vi "TDMS to ASCII convertor.vi"(8 "error in":errorcluster, 9 "Group handling":enum16{"One file per group", "Ignore groups"}(ring), 11 "TDMS file path":path) -> (0 "error out":errorcluster, 3 "Generated File Path(s)":path[](array[path]))   [LabVIEW 2016]
uses:
  <vilib>/Utility/file.llb/Write To Spreadsheet File (string).vi
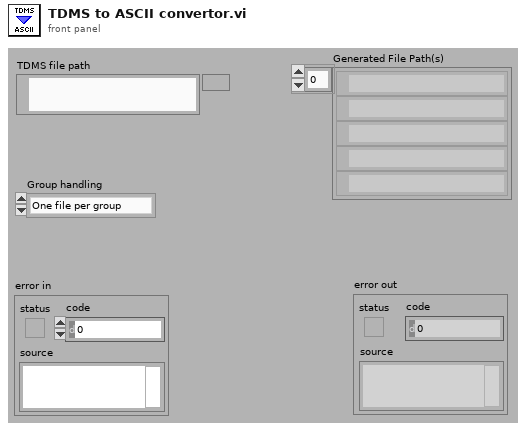
[diagram p1: front panel]
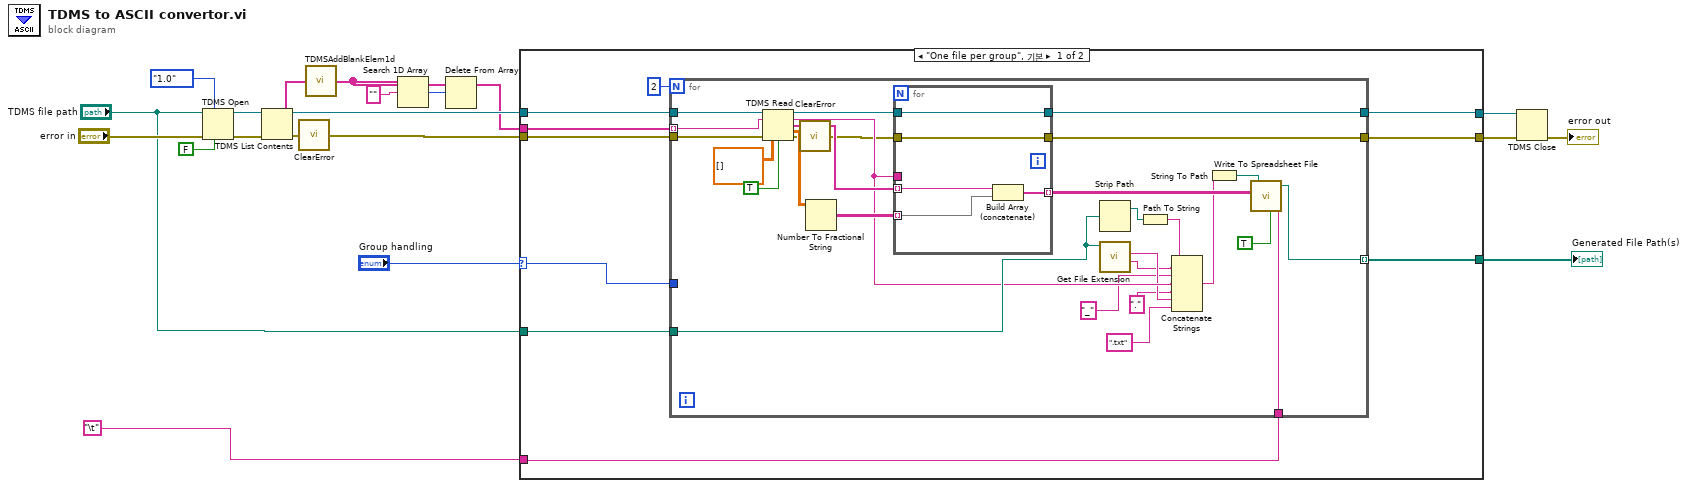
[diagram p0: block diagram]
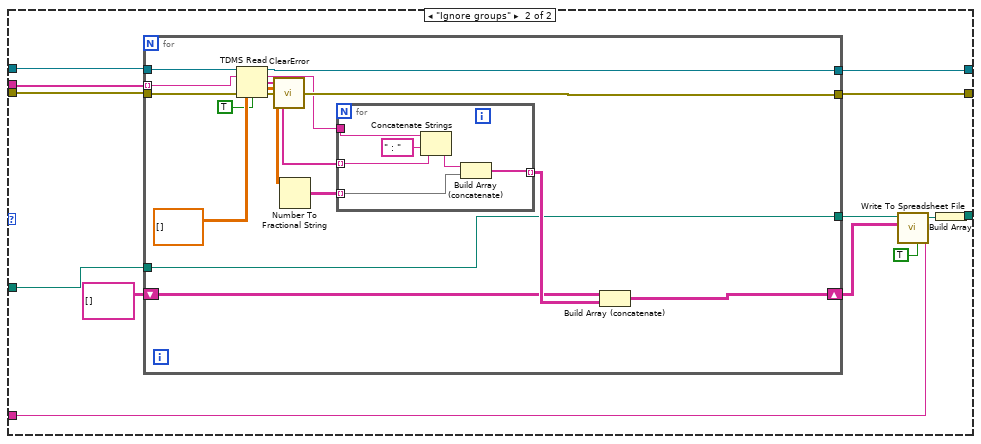
[diagram p2: hidden frame]
diagram:
  n1 = TDMS Open(6:FALSE ("버퍼링 비활성화? (참)"), 7:enum16{"1.0", "2.0"}."1.0" ("파일 포맷 버전(2.0)"), 8:"error in", 11:"TDMS file path") -> (0:w17:errorcluster, 3:w18:refnum<k34>)  [unwired: 3 in]
  n2 = TDMS List Contents(4:w17, 7:w18) -> (0:w1:errorcluster, 2:w4:string[], 3:w16:refnum<k34>)  [unwired: 1 in, 1 out]
  n3 = call <vilib>:"ClearError.vi"("error in (no error)"=w1) -> ("error out"=w15:errorcluster)
  n4 = call <vilib>:"TDMSAddBlankElem1d.vi"("input string array"=w4) -> ("output string array with blank element at the beginning"=w9:string[])
  n5 = Search 1D Array(1D array=w9, element="") -> (index of element=w7:i32)  [unwired: 1 in]
  n6 = Delete From Array(array=w9, index=w7) -> (array with subset deleted=w14:string[])  [unwired: 1 in, 1 out]
  n7 = case shown="\"One file per group\", 기본" "Group handling" {
    selector: "Group handling" -> [w29 _]
    tunnel: "TDMS file path" -> [w30 w73]
    tunnel: [w28 w68] -> w19
    tunnel: w16 -> [w24 w76]
    tunnel: w14 -> [w27 w75]
    tunnel: w15 -> [w26 w74]
    tunnel: [w23 w67] -> w13
    tunnel: [w22 w66] -> w12
    tunnel: "\t" -> [w25 w64]
    frame "One file per group", Default {
      n8 = for {
        N: 2 -> [_]
        tunnel: w30 -> [w58]
        tunnel: w26 -> [w54]
        tunnel: w24 -> [w53]
        tunnel: w27 -> [w36] mode=indexing
        tunnel: w29 -> [_]
        tunnel: [w52] -> w28 mode=indexing
        tunnel: w25 -> [w39]
        tunnel: [w35] -> w23
        tunnel: [w34] -> w22
        n9 = TDMS Read(0:w53, 5:w36, 11:w54, 12:dbl[][] [] ("channel name(s) out"), 13:TRUE ("파일 순서로 채널 반환? (거짓)")) -> (4:w38:refnum<k34>, 6:w49:string, 8:w56:string[], 10:w55:dbl[][], 15:w32:errorcluster)  [unwired: 3 in, 1 out]
        n10 = call <vilib>:"ClearError.vi"("error in (no error)"=w32) -> ("error out"=w37:errorcluster)
        n11 = Number To Fractional String(number=w55) -> (F-format string=w51:string[][])  [unwired: 3 in]
        n12 = for {
          tunnel: w56 -> [w61] mode=indexing
          tunnel: [w63] -> w50 mode=indexing
          tunnel: w51 -> [w62] mode=indexing
          tunnel: w49 -> [_]
          tunnel: w38 -> [w60]
          tunnel: w37 -> [w59]
          tunnel: [w60] -> w35
          tunnel: [w59] -> w34
          n13 = Build Array (concatenate)(w61, w62) -> (w63:string[])
        }
        n14 = Strip Path(path=w58) -> (stripped path=w43:path)  [unwired: 1 out]
        n15 = call <vilib>:"Get File Extension.vi"("file"=w58) -> ("filename without extension"=w45:string, "lowercase file extension"=w48:string)  [unwired: 6 in, 3 out]
        n16 = Path To String(path=w43) -> (string=w42:string)
        n17 = Concatenate Strings(w42, w45, "_" ("delimiter (\\t)"), w49, "." ("delimiter (\\t)"), w48, ".txt" ("문자열")) -> (w44:string)
        n18 = String To Path(string=w44) -> (path=w40:path)
        n19 = call-poly <vilib>:"Write To Spreadsheet File.vi"("delimiter (\\t)"=w39, "transpose? (no:F)"=TRUE, "2D data"=w50, "file path (dialog if empty)"=w40) -> ("new file path (Not A Path if cancelled)"=w52:path)  [unwired: 4 in]
      }
    }
    frame "Ignore groups" {
      n20 = for {
        tunnel: [w92] -> w67
        tunnel: w73 -> [w79]
        tunnel: w74 -> [w88]
        tunnel: [w87] -> w66
        tunnel: w76 -> [w86]
        tunnel: w75 -> [w85] mode=indexing
        tunnel: [w79] -> w71
        shift-right: [w82] -> w70
        shift-left: string[][] [] -> [w80]
        n21 = TDMS Read(0:w86, 5:w85, 11:w88, 12:dbl[][] [] ("channel name(s) out"), 13:TRUE ("파일 순서로 채널 반환? (거짓)")) -> (4:w92:refnum<k34>, 6:w83:string, 8:w90:string[], 10:w89:dbl[][], 15:w77:errorcluster)  [unwired: 3 in, 1 out]
        n22 = call <vilib>:"ClearError.vi"("error in (no error)"=w77) -> ("error out"=w87:errorcluster)
        n23 = Number To Fractional String(number=w89) -> (F-format string=w84:string[][])  [unwired: 3 in]
        n24 = for {
          tunnel: w90 -> [w95] mode=indexing
          tunnel: [w98] -> w81 mode=indexing
          tunnel: w84 -> [w97] mode=indexing
          tunnel: w83 -> [w93]
          n25 = Concatenate Strings(w93, " : " ("element"), w95) -> (w96:string)
          n26 = Build Array (concatenate)(w96, w97) -> (w98:string[])
        }
        n27 = Build Array (concatenate)(w80, w81) -> (w82:string[][])
      }
      n28 = call-poly <vilib>:"Write To Spreadsheet File.vi"("delimiter (\\t)"=w64, "transpose? (no:F)"=TRUE, "2D data"=w70, "file path (dialog if empty)"=w71) -> ("new file path (Not A Path if cancelled)"=w69:path)  [unwired: 4 in]
      n29 = Build Array(w69) -> (w68:path[])
    }
  }
  "Generated File Path(s)" <- w19
  n30 = TDMS Close(8:w12, 11:w13) -> (0:→"error out":errorcluster)  [unwired: 1 out]
